vi "FTW-Actor-InitializeLocalMessageWorkers.vi"(0 "FTW Actor Instance Type":refnum<class "FTW-ActorInstance.lvclass">, 7 "Actor Instance Configuration":string, 11 "error in":errorcluster) -> (4 "FTW Actor Instance":refnum<class "FTW-ActorInstance.lvclass">, 15 "error out":errorcluster)   [LabVIEW 2018, in "FTW-ActorInstance.lvclass"]
uses:
  FTW-ActorInstance.lvclass
  705bac67-a62c-4146-90a6-c3ed0fe53033.vi
  FTW-Actor-LocalMessage-Worker.vi
  JSON/core/FTW-JSON-Core-EncodingFlags.vi
  Reflection/FTW-Reflection-Type.vi
  JSON/FTW-JSON-Parse.vi
  container/FTW-Container-GetFlattenedValue.vi
panel:
  # "Inputs"
  # "Outputs"
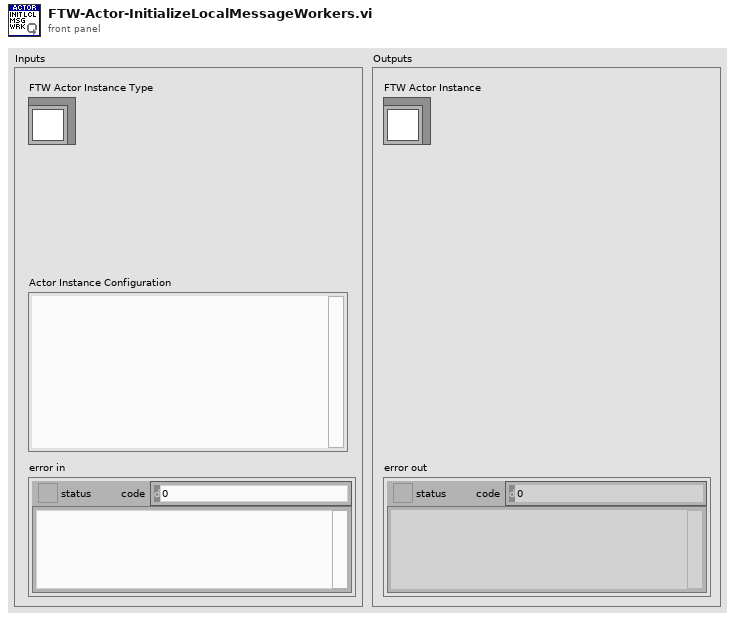
[diagram p1: front panel]
types:
  T1 = cluster{"MessageBody":string, "SendRate":dbl, "Lossless":bool, "MaxQueueSize":i32}
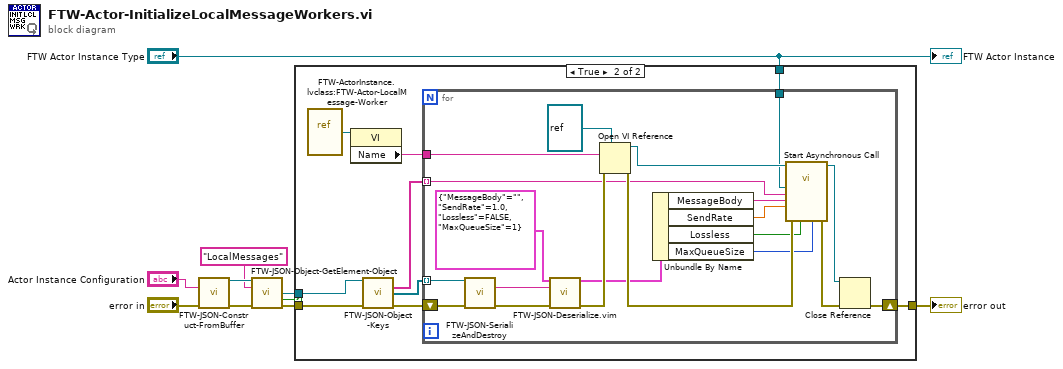
[diagram p0: block diagram]
diagram:
  n1 = call "FTW-JSON-Construct-FromBuffer.vi"("JSON String (UTF-8)"="Actor Instance Configuration", "error in"="error in") -> ("JSON"=w5:refnum<class "FTW-Container.lvclass">, "error out"=w8:errorcluster)  [unwired: 12 in]
  n2 = call "FTW-JSON-Object-GetElement-Object.vi"("JSON"=w5, "Key"="LocalMessages", "error in"=w8) -> ("Value"=w3:refnum<class "FTW-Container.lvclass">, "Found"=w1:bool, "error out"=w6:errorcluster)  [unwired: 8 in, 2 out]
  n3 = case shown="True" w1 {
    tunnel: [w11 w18] -> w10
    tunnel: w6 -> [w11 w17]
    tunnel: w3 -> [_ w15]
    tunnel: "FTW Actor Instance Type" -> [_ w14]
    frame False {
    }
    frame True {
      n4 = vi-ref "FTW-ActorInstance.lvclass:FTW-Actor-LocalMessage-Worker.vi"() -> (w20:refnum<vi>)
      n5 = property class="VI"(reference=w20) -> ("Name"=w19:string)  [unwired: 1 in, 2 out]
      n6 = call "FTW-JSON-Object-Keys.vi"("FTW-Container In"=w15, "error in"=w17) -> ("Object Keys"=w12:string[], "Object Elements"=w13:refnum<class "FTW-Container.lvclass">[], "error out"=w16:errorcluster)  [unwired: 10 in, 1 out]
      n7 = for {
        tunnel: w19 -> [w35]
        tunnel: w14 -> [w32]
        shift-right: [w33] -> w18
        shift-left: w16 -> [w30]
        tunnel: w13 -> [w27] mode=indexing
        tunnel: w12 -> [w31] mode=indexing
        n8 = call "FTW-JSON-SerializeAndDestroy.vi"("JSON"=w27, "error in"=w30) -> ("JSON String (UTF-8)"=w26:string, "error out"=w28:errorcluster)  [unwired: 12 in]
        n9 = call "FTW-JSON-Deserialize.vim"("Type In"=T1 {"MessageBody"="", "SendRate"=1.0, "Lossless"=FALSE, "MaxQueueSize"=1}, "JSON String"=w26, "error in"=w28) -> ("Type Out"=w25:T1, "error out"=w38:errorcluster)  [unwired: 11 in]
        n10 = Open VI Reference(type specifier VI Refnum (for type only)=refnum<vi> refnum, vi path=w35, error in (no error)=w38) -> (vi reference=w37:refnum<vi>, error out=w40:errorcluster)  [unwired: 3 in]
        n11 = Unbundle By Name(w25) -> ("MessageBody"=w24:string, "SendRate"=w23:dbl, "Lossless"=w22:bool, "MaxQueueSize"=w21:i32)
        n12 = call-by-ref "Start Asynchronous Call"(reference=w37, error in=w40, "FTW-ActorInstance In"=w32, "Message Header"=w31, "Message Body"=w24, "Send Rate"=w23, "Lossless (F)"=w22, "max queue size (1)"=w21) -> (reference out=w34:refnum<vi>, error out=w39:errorcluster)  [unwired: 10 in]
        n13 = Close Reference(reference=w34, error in (no error)=w39) -> (error out=w33:errorcluster)
      }
    }
  }
  "error out" <- w10
  "FTW Actor Instance" <- "FTW Actor Instance Type"
